vi "Read CR5.vi"(8 "error in (no error)":errorcluster, 11 "tCRD in":refnum<class "Open Path CRD.lvclass">) -> (0 "error out":errorcluster, 2 "CR5":refnum<class "CR5.lvclass">, 3 "tCRD out":refnum<class "Open Path CRD.lvclass">)   [LabVIEW 2015, in "Open Path CRD.lvclass"]
uses:
  Open Path CRD.lvclass
  Devices/CR5/CR5.lvclass
  Open Path CRD.lvclass/Open Path CRD.ctl
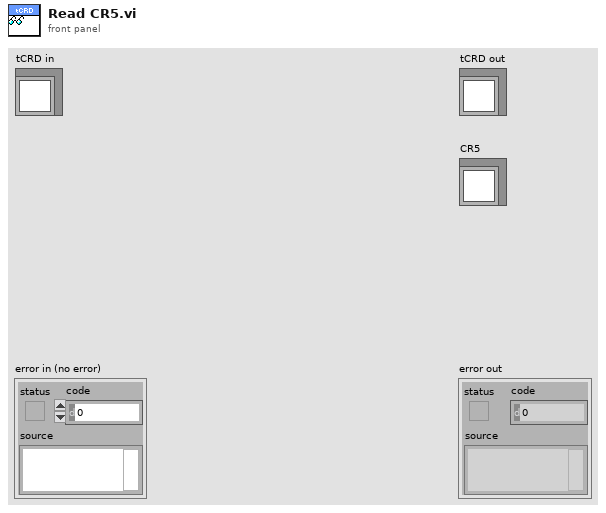
[diagram p1: front panel]
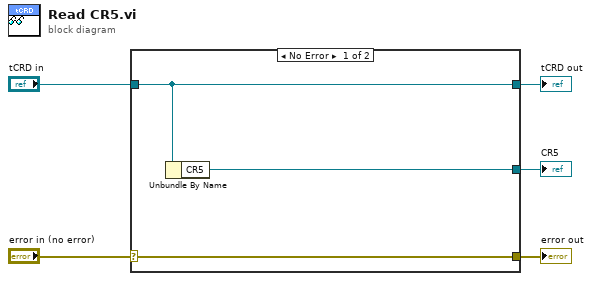
[diagram p0: block diagram]
diagram:
  n1 = case shown="No Error" "error in (no error)" {
    selector: "error in (no error)" -> [w8 w9]
    tunnel: [w8 w9] -> w4
    tunnel: [w7 w10] -> w2
    tunnel: "tCRD in" -> [w7 w10]
    tunnel: [w6 _] -> w1
    frame No Error {
      n2 = Unbundle By Name(w7) -> ("CR5"=w6:refnum<class "CR5.lvclass">)
    }
    frame Error {
    }
  }
  "error out" <- w4
  "tCRD out" <- w2
  "CR5" <- w1
